vi "Calc Type.vi"(11 "Tare Calc in":refnum<class "Tare Calc.lvclass">) -> (2 "Calc Type":string)   [LabVIEW 2020, in "VolatusCalcs.lvlib" / "Tare Calc.lvclass"]
uses:
  Tare Calc.lvclass
  Tare Calc.lvclass/Tare Calc.ctl
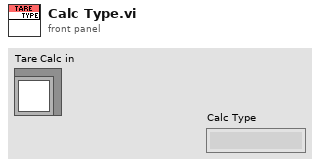
[diagram p1: front panel]
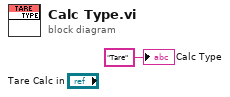
[diagram p0: block diagram]
diagram:
  "Calc Type" <- "Tare" ("Calc Type")
